vi "I2C_read.vi"(8 "error in (no error)":errorcluster, 10 "Combo Box":string(combo)) -> (0 "error out":errorcluster, 2 "x/y":dbl format="%#_5g")   [LabVIEW 2023]
panel:
  out "Hex string":string
  out "CMD output":string
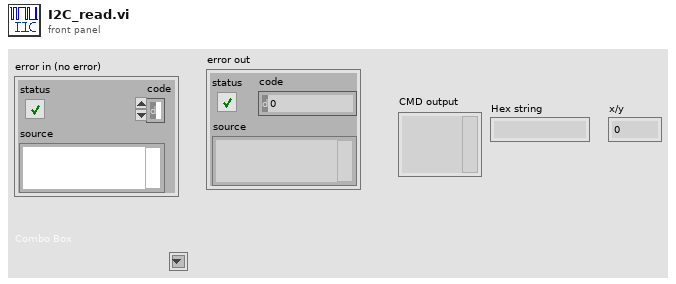
[diagram p1: front panel]
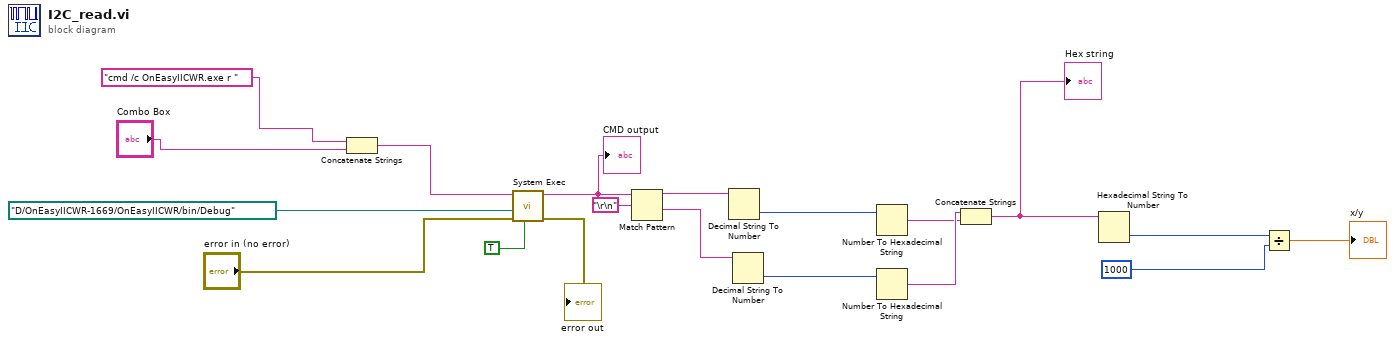
[diagram p0: block diagram]
diagram:
  n1 = Concatenate Strings("cmd /c OnEasyIICWR.exe r " ("command line"), "Combo Box") -> (w3:string)
  n2 = call <vilib>:"System Exec.vi"("run minimized? (F)"=TRUE, "error in (no error)"="error in (no error)", "working directory"=path "D:/OnEasyIICWR-1669/OnEasyIICWR/bin/Debug", "command line"=w3) -> ("error out"=→"error out":errorcluster, "standard output"=w17:string)  [unwired: 4 in, 2 out]
  "CMD output" <- w17
  n3 = Match Pattern(string=w17, regular expression="\r\n") -> (before substring=w15:string, after substring=w12:string)  [unwired: 1 in, 2 out]
  n4 = Decimal String To Number(string=w15) -> (number=w14:i32)  [unwired: 2 in, 1 out]
  n5 = Decimal String To Number(string=w12) -> (number=w13:i32)  [unwired: 2 in, 1 out]
  n6 = Number To Hexadecimal String(2:w14) -> (0:w10:string)  [unwired: 1 in]
  n7 = Number To Hexadecimal String(2:w13) -> (0:w11:string)  [unwired: 1 in]
  n8 = Concatenate Strings(w11, w10) -> (w9:string)
  "Hex string" <- w9
  n9 = Hexadecimal String To Number(string=w9) -> (number=w8:u32)  [unwired: 2 in, 1 out]
  n10 = Divide(x=w8, y=u32 1000) -> (x/y=→"x/y":dbl)
